vi "DAC Configure.vi"(8 "error in":errorcluster, 11 "DAC Pressure Scan in":refnum<class "DAC Pressure Scan.lvclass">) -> (0 "error out":errorcluster, 3 "DAC Pressure Scan out":refnum<class "DAC Pressure Scan.lvclass">)   [LabVIEW 2019, in "DAC.lvlib" / "DAC Pressure Scan.lvclass"]
uses:
  DAC Pressure Scan.lvclass
  C:/Users/wg/Documents/LV_Projects/test-stand/App/DAC/DAC.lvclass
  DAC.lvclass/DAC.ctl
  DAC Pressure Scan.lvclass/DAC Pressure Scan.ctl
  <vilib>/DAQmx/create/channels.llb/DAQmx Create Channel (AI-Voltage-Basic).vi
  DAC.lvclass
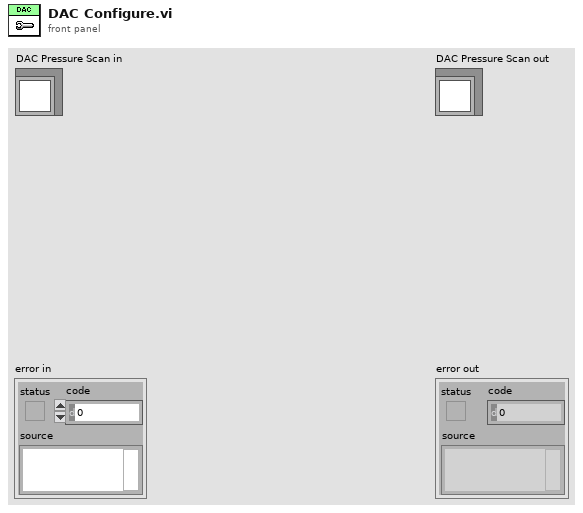
[diagram p1: front panel]
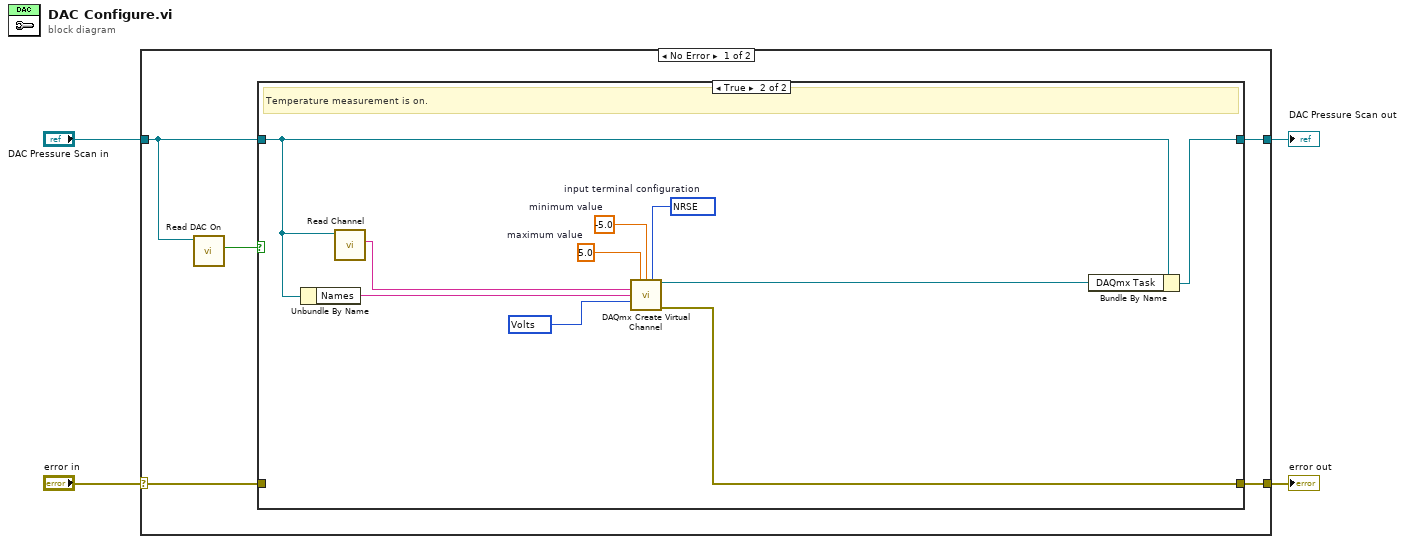
[diagram p0: block diagram]
diagram:
  n1 = case shown="No Error" "error in" {
    selector: "error in" -> [w6 w23]
    tunnel: [w5 w23] -> w4
    tunnel: [w7 w22] -> w3
    tunnel: "DAC Pressure Scan in" -> [w9 w22]
    frame No Error {
      n2 = call "Read DAC On.vi"("DAC in"=w9) -> ("DAC On"=w8:bool)  [unwired: 8 in, 2 out]
      n3 = case shown="True" w8 {
        tunnel: w9 -> [w11 w13]
        tunnel: [w11 w21] -> w7
        tunnel: w6 -> [w10 _]
        tunnel: [w10 w20] -> w5
        frame False {
          # "Temperature measurement is off."
        }
        frame True {
          w14 = 5.0  # maximum value
          w15 = -5.0  # minimum value
          w16 = 10078 items=["Default"=-1, "RSE"=10083, "NRSE"=10078, "Differential"=10106, "Pseudodifferential"=12529]  # input terminal configuration
          w17 = 10348 items=["Volts"=10348, "From Custom Scale"=10065] ("units")
          # "Temperature measurement is on."
          n4 = Unbundle By Name(w13) -> ("Names"=w19:string)
          n5 = call "Read Channel.vi"("DAC in"=w13) -> ("Channel"=w12:string)  [unwired: 8 in, 2 out]
          n6 = call-poly <vilib>:"DAQmx Create Virtual Channel.vi"("maximum value"=w14, "minimum value"=w15, "input terminal configuration"=w16, "physical channels"=w12, "name to assign"=w19, "units"=w17) -> ("task out"=w18:refnum<k21>, "error out"=w20:errorcluster)  [unwired: 8 in]
          n7 = Bundle By Name(cluster=w13, "DAQmx Task"=w18) -> (w21:refnum<class "DAC Pressure Scan.lvclass">)
        }
      }
    }
    frame Error {
    }
  }
  "error out" <- w4
  "DAC Pressure Scan out" <- w3
